vi "Is Attached To Node.vi"(0 "FSM.Edge In":refnum<class "FSM.Edge.lvclass">, 7 "nodeName":string) -> (4 "FSM.Edge Out":refnum<class "FSM.Edge.lvclass">, 8 "attached to":bool)   [LabVIEW 2020, in "FSM.Edge.lvclass"]
uses:
  FSM.Edge.lvclass
  FSM.Edge.lvclass/FSM.Edge.ctl
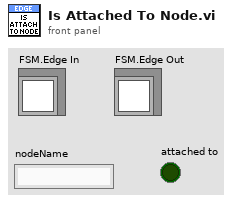
[diagram p1: front panel]
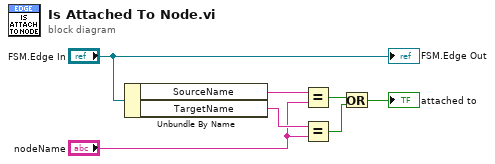
[diagram p0: block diagram]
diagram:
  n1 = Unbundle By Name("FSM.Edge In") -> ("SourceName"=w7:string, "TargetName"=w6:string)
  n2 = Equal?(x=w7, y="nodeName") -> (x = y?=w4:bool)
  n3 = Equal?(x=w6, y="nodeName") -> (x = y?=w3:bool)
  n4 = Or(x=w4, y=w3) -> (x .or. y?=→"attached to":bool)
  "FSM.Edge Out" <- "FSM.Edge In"
